vi "FindNearestElement.vi"(8 "Starting Index":i32, 9 "Desired Element":dbl, 11 "Input Array":dbl[](array[numeric])) -> (0 "Closest Index":i32, 2 "Closest Element":dbl)   [LabVIEW 2019]
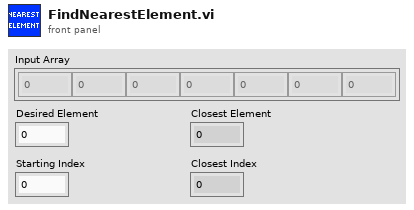
[diagram p1: front panel]
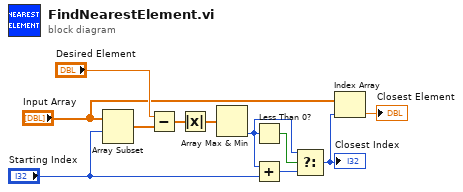
[diagram p0: block diagram]
diagram:
  n1 = Array Subset(array="Input Array", index="Starting Index") -> (w9:dbl[])  [unwired: 1 in]
  n2 = Subtract(x="Desired Element", y=w9) -> (x-y=w10:dbl[])
  n3 = Absolute Value(x=w10) -> (abs(x)=w11:dbl[])
  n4 = Array Max & Min(array=w11) -> (min index (indices)=w5:i32)  [unwired: 3 out]
  n5 = Less Than 0?(x=w5) -> (x < 0?=w4:bool)
  n6 = Add(x=w5, y="Starting Index") -> (x+y=w6:i32)
  n7 = Select(t=w5, s=w4, f=w6) -> (s? t:f=w3:i32)
  "Closest Index" <- w3
  n8 = Index Array(array="Input Array", index=w3) -> (element=→"Closest Element":dbl)
